vi "Result_Test.vi"(8 "error in (no error)":errorcluster caption="entrée d'erreur (pas d'erreur)", 11 "Get_Voltage en entrée":refnum<class "Read_Frequency.lvclass">) -> (0 "error out":errorcluster caption="sortie d'erreur", 3 "Get_Voltage en sortie":refnum<class "Read_Frequency.lvclass">)   [LabVIEW 2020, in "Library Test.lvlib" / "Read_Frequency.lvclass"]
uses:
  Read_Frequency.lvclass
  C:/Users/ngarcin/OneDrive - Altyor/Standard TB/Class/Test/Test (Default)/Test (Default).lvclass
  JSON API/JSON Value/Set from JSON string.vi
  Instrument/Instrument (Default)/Class Instrument (Default).lvclass
  JSON API/JSON Value/JSON Value.lvclass
  Read_Spectrum_Analyser/Read_Spectrum_Analyser.lvclass
  Read_Frequency.lvclass/Read_Frequency.ctl
  JSON API/Variant JSON/Variant JSON.lvlib
  JSON API/Get Polymorphic/JSON GetSet.lvlib
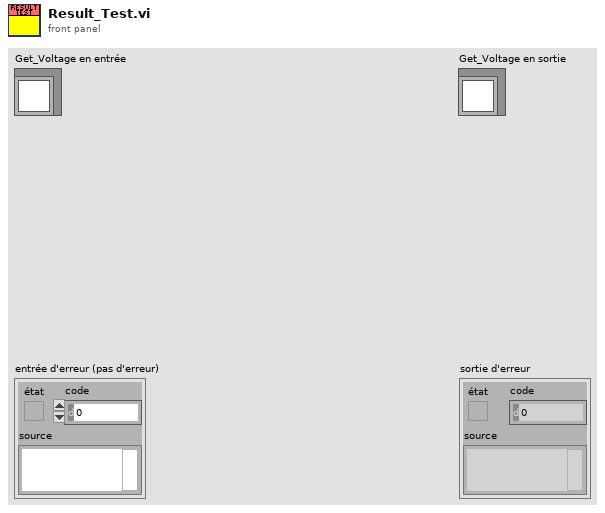
[diagram p1: front panel]
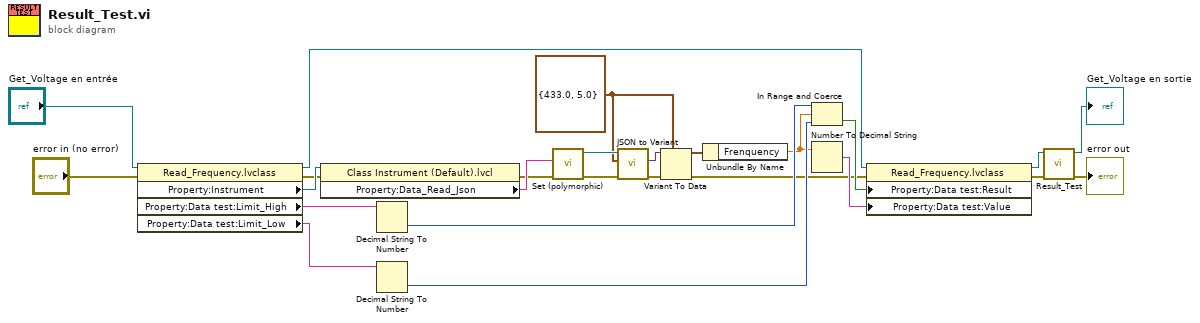
[diagram p0: block diagram]
diagram:
  w1 = cluster{"Frenquency":dbl, "Power":dbl} {"Frenquency"=433.0, "Power"=5.0} ("Parameter")
  n1 = property class="Read_Frequency.lvclass"(reference="Get_Voltage en entrée", error in="error in (no error)") -> (reference out=w16:refnum<class "Read_Frequency.lvclass">, error out=w3:errorcluster, "Property:Instrument"=w5:refnum<class "Class Instrument (Default).lvclass">, "Property:Data test:Limit_High"=w15:string, "Property:Data test:Limit_Low"=w14:string)
  n2 = property class="Class Instrument (Default).lvcl"(reference=w5, error in=w3) -> (error out=w2:errorcluster, "Property:Data_Read_Json"=w4:string)  [unwired: 1 out]
  n3 = Decimal String To Number(string=w15) -> (number=w13:i32)  [unwired: 2 in, 1 out]
  n4 = Decimal String To Number(string=w14) -> (number=w12:i32)  [unwired: 2 in, 1 out]
  n5 = call-poly "Set (polymorphic).vi"("error in (no error)"=w2, "JSON stream"=w4) -> ("error out"=w21:errorcluster, "JSON Value out"=w19:refnum<class "JSON Value.lvclass">)  [unwired: 7 in, 1 out]
  n6 = call "JSON to Variant.vi"("error in (no error)"=w21, "Variant (Data Type)"=w1, "JSON Value"=w19) -> ("error out"=w20:errorcluster, "Variant out"=w18:variant)  [unwired: 7 in]
  n7 = Variant To Data(error in=w20, type=w1, Variant=w18) -> (data=w17:cluster{"Frenquency":dbl, "Power":dbl}, error out=w8:errorcluster)
  n8 = Unbundle By Name(w17) -> ("Frenquency"=w10:dbl)
  n9 = In Range and Coerce(upper limit=w13, x=w10, lower limit=w12) -> (In Range?=w11:bool)  [unwired: 1 out]
  n10 = Number To Decimal String(number=w10) -> (decimal integer string=w9:string)  [unwired: 1 in]
  n11 = property class="Read_Frequency.lvclass"(reference=w16, error in=w8, "Property:Data test:Result"=w11, "Property:Data test:Value"=w9) -> (reference out=w7:refnum<class "Read_Frequency.lvclass">, error out=w6:errorcluster)
  n12 = call-parent "Result_Test.vi"("error in (no error)"=w6, "Get_Voltage en entrée"=w7) -> ("error out"=→"error out":errorcluster, "Get_Voltage en sortie"=→"Get_Voltage en sortie":refnum<class "Read_Frequency.lvclass">)  [unwired: 8 in]
